vi "GITChangedFiles.vi"(8 "error in":errorcluster, 10 "RepoRoot":path, 11 "Remote Branch to Compare":string="develop") -> (0 "error out":errorcluster, 2 "Files Changed":path[](array[path]))   [LabVIEW 2020, in "CICD.lvlib"]
doc: "Compares the current branch to the specified remote branch and returns a list of all file changes in the current branch."
uses:
  CICD.lvlib
panel:
  out "standard output":string
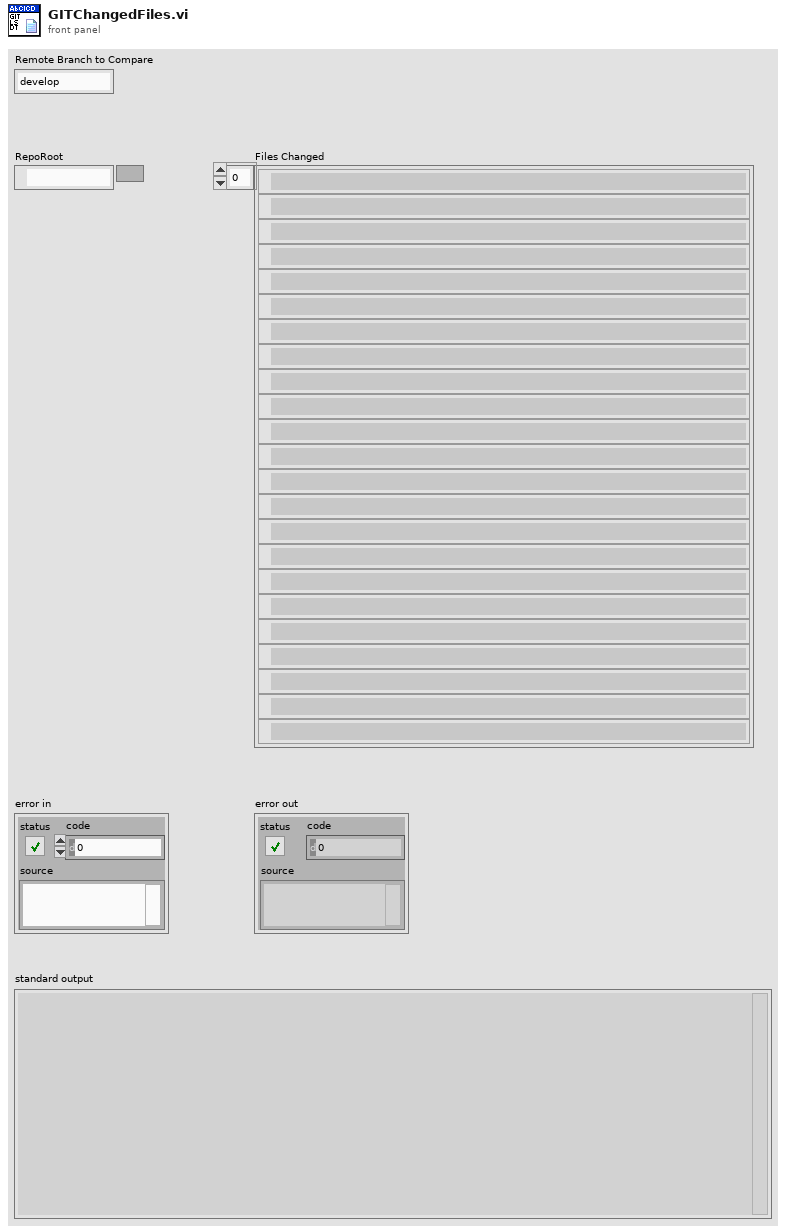
[diagram p1: front panel]
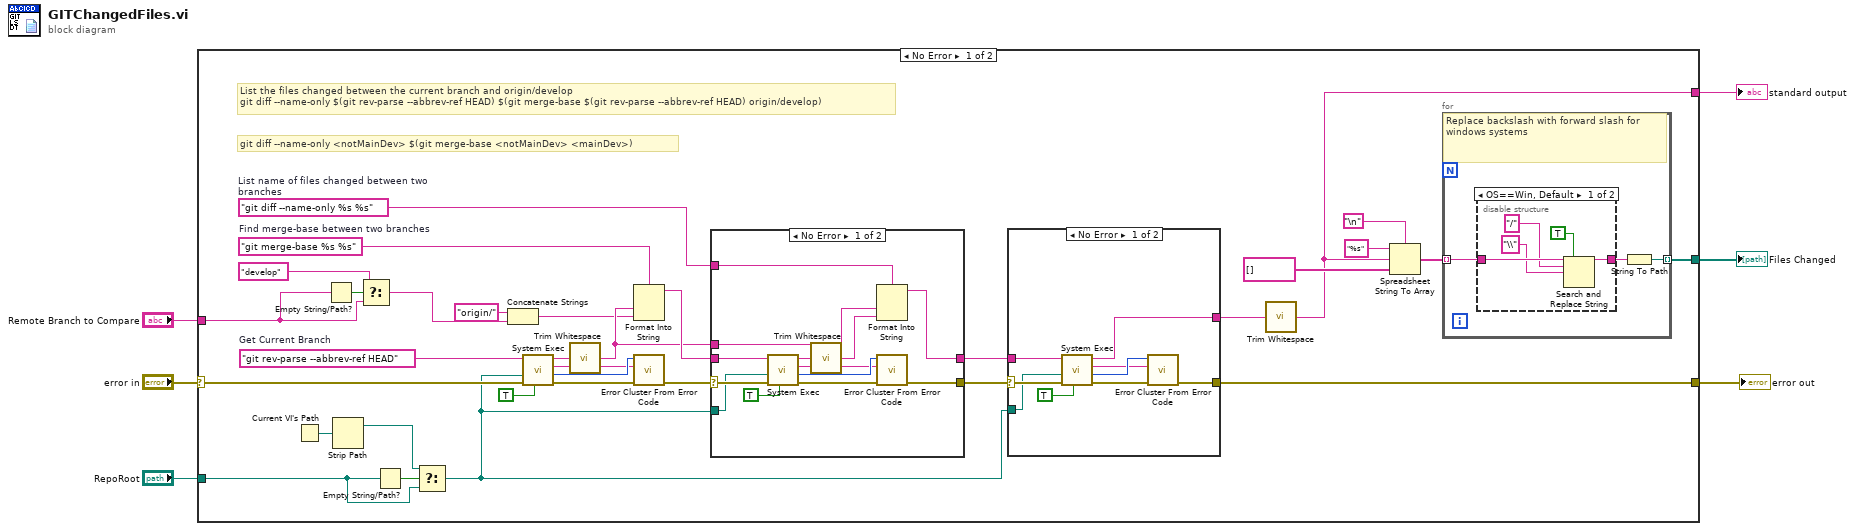
[diagram p0: block diagram]
diagram:
  n1 = case shown="No Error" "error in" {
    selector: "error in" -> [w35 w75]
    tunnel: [w38 w75] -> w6
    tunnel: [w23 _] -> w4
    tunnel: [w18 _] -> w3
    tunnel: "Remote Branch to Compare" -> [w15 _]
    tunnel: "RepoRoot" -> [w8 _]
    frame No Error {
      w33 = "git merge-base %s %s"  # Find merge-base between two branches
      w30 = "git diff --name-only %s %s"  # List name of files changed between two branches
      w34 = "git rev-parse --abbrev-ref HEAD"  # Get Current Branch
      # "List the files changed between the current branch and origin/develop\ngit diff --name-only $(git rev-parse --abbrev-ref HEAD) $(git merge-base $(git rev-parse --abbrev-ref HEAD) origin/develop)"
      # "git diff --name-only <notMainDev> $(git merge-base <notMainDev> <mainDev>)"
      n2 = Current VI's Path() -> (path=w12:path)
      n3 = Empty String/Path?(string/path=w15) -> (empty?=w16:bool)
      n4 = Strip Path(path=w12) -> (stripped path=w10:path)  [unwired: 1 out]
      n5 = Select(t="develop", s=w16, f=w15) -> (s? t:f=w14:string)
      n6 = Empty String/Path?(string/path=w8) -> (empty?=w11:bool)
      n7 = Select(t=w10, s=w11, f=w8) -> (s? t:f=w9:path)
      n8 = Concatenate Strings("origin/" ("string"), w14) -> (w17:string)
      n9 = call <vilib>:"System Exec.vi"("run minimized? (F)"=TRUE, "error in (no error)"=w35, "working directory"=w9, "command line"=w34) -> ("error out"=w39:errorcluster, "return code"=w21:i32, "standard error"=w20:string, "standard output"=w28:string)  [unwired: 4 in]
      n10 = call <vilib>:"Trim Whitespace.vi"("string"=w28) -> ("trimmed string"=w27:string)  [unwired: 1 in]
      n11 = Format Into String(format string=w33, w27, w17) -> (resulting string=w32:string)  [unwired: 2 in, 1 out]
      n12 = call <vilib>:"Error Cluster From Error Code.vi"("error in (no error)"=w39, "error message (\"\")"=w20, "error code (0)"=w21) -> ("error out"=w37:errorcluster)  [unwired: 6 in]
      n13 = case shown="No Error" w37 {
        selector: w37 -> [w70 w74]
        tunnel: w32 -> [w69 _]
        tunnel: w30 -> [w68 _]
        tunnel: [w67 w73] -> w29
        tunnel: w27 -> [w65 w73]
        tunnel: [w71 w74] -> w36
        tunnel: w9 -> [w60 _]
        frame No Error {
          n14 = call <vilib>:"System Exec.vi"("run minimized? (F)"=TRUE, "error in (no error)"=w70, "working directory"=w60, "command line"=w69) -> ("error out"=w72:errorcluster, "return code"=w63:i32, "standard error"=w62:string, "standard output"=w66:string)  [unwired: 4 in]
          n15 = call <vilib>:"Trim Whitespace.vi"("string"=w66) -> ("trimmed string"=w64:string)  [unwired: 1 in]
          n16 = Format Into String(format string=w68, w65, w64) -> (resulting string=w67:string)  [unwired: 2 in, 1 out]
          n17 = call <vilib>:"Error Cluster From Error Code.vi"("error in (no error)"=w72, "error message (\"\")"=w62, "error code (0)"=w63) -> ("error out"=w71:errorcluster)  [unwired: 6 in]
        }
        frame Error {
        }
      }
      n18 = case shown="No Error" w36 {
        selector: w36 -> [w55 w59]
        tunnel: [w54 w58] -> w31
        tunnel: w29 -> [w53 w58]
        tunnel: [w56 w59] -> w38
        tunnel: w9 -> [w49 _]
        frame No Error {
          n19 = call <vilib>:"System Exec.vi"("run minimized? (F)"=TRUE, "error in (no error)"=w55, "working directory"=w49, "command line"=w53) -> ("error out"=w57:errorcluster, "return code"=w52:i32, "standard error"=w51:string, "standard output"=w54:string)  [unwired: 4 in]
          n20 = call <vilib>:"Error Cluster From Error Code.vi"("error in (no error)"=w57, "error message (\"\")"=w51, "error code (0)"=w52) -> ("error out"=w56:errorcluster)  [unwired: 6 in]
        }
        frame Error {
        }
      }
      n21 = call <vilib>:"Trim Whitespace.vi"("string"=w31) -> ("trimmed string"=w23:string)  [unwired: 1 in]
      n22 = Spreadsheet String To Array(delimiter (Tab)="\n", format string="%s", spreadsheet string=w23, array type (2D Dbl)=string[] []) -> (array=w24:string[])
      n23 = for {
        tunnel: w24 -> [w42] mode=indexing
        tunnel: [w40] -> w18 mode=indexing
        # "Replace backslash with forward slash for windows systems"
        n24 = disable-structure shown="OS==Win, Default" {
          disable-tunnel: w42 -> [w47 w48]
          disable-tunnel: [w46 w48] -> w41
          frame condition #0 (active) {
            n25 = Search and Replace String(replace all?=TRUE ("replace all? (F)"), input string=w47, search string="/", replace string="\\" ("search string")) -> (result string=w46:string)  [unwired: 4 in, 3 out]
          }
          frame condition #1 {
          }
        }
        n26 = String To Path(string=w41) -> (path=w40:path)
      }
    }
    frame Error {
    }
  }
  "error out" <- w6
  "standard output" <- w4
  "Files Changed" <- w3
